vi "Mutate 1-0-4-11.vi"(8 "error in (no error)":errorcluster, 11 "Device Ref in":T1 format="%.0x") -> (0 "error out":errorcluster, 2 "New CD Version":string="1.0.2.2", 3 "Device Ref out":T1 format="%.0x")   [LabVIEW 2021, in "G5 Regatron Custom Device System Explorer.lvlib"]
uses:
  G5 Regatron Custom Device System Explorer.lvlib
  <vilib>/NI VeriStand/Custom Device API/Custom Device Item Ref.ctl
  <vilib>/NI VeriStand/Custom Device API/Custom Device API.lvlib
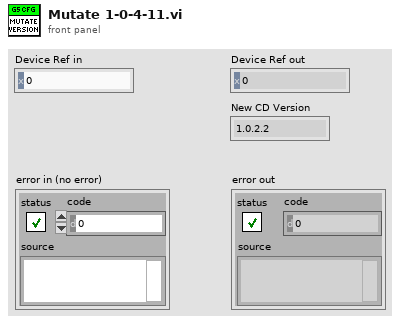
[diagram p1: front panel]
types:
  T1 = typedef "Custom Device API.lvlib/Custom Device Item Ref.ctl" = u64
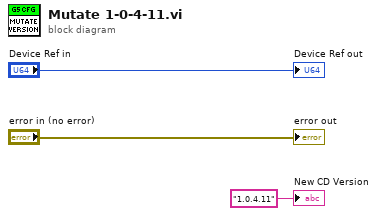
[diagram p0: block diagram]
diagram:
  "error out" <- "error in (no error)"
  "Device Ref out" <- "Device Ref in"
  "New CD Version" <- "1.0.4.11"
